vi "exec.vi"(8 "error in (no error)":errorcluster, 10 "context":refnum<class "IContextThisComponent.lvclass">, 11 "ClearError in":refnum<class "ClearError.lvclass">) -> (0 "error out":errorcluster, 2 "context 2":refnum<class "IContextThisComponent.lvclass">, 3 "ClearError out":refnum<class "ClearError.lvclass">)   [LabVIEW 2012, in "Commands.lvlib" / "ClearError.lvclass"]
uses:
  ClearError.lvclass
  IContextThisComponent/IContextThisComponent.lvclass
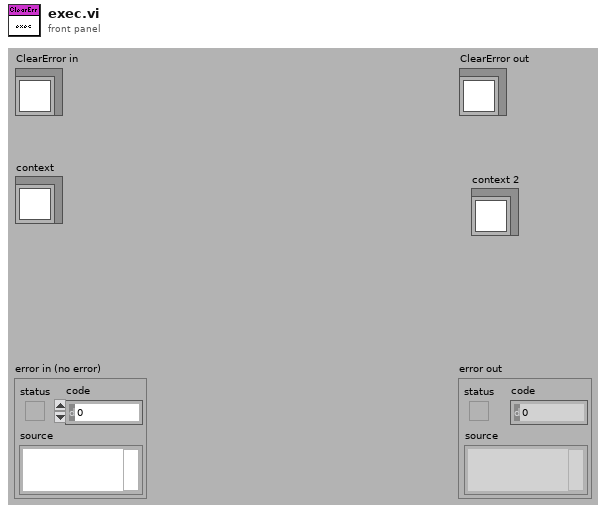
[diagram p1: front panel]
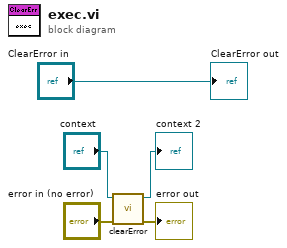
[diagram p0: block diagram]
diagram:
  n1 = call-dynamic "clearError.vi"("error in (no error)"="error in (no error)", "IContextThisComponent in"="context") -> ("error out"=→"error out":errorcluster, "IContextThisComponent out"=→"context 2":refnum<class "IContextThisComponent.lvclass">)  [unwired: 8 in]
  "ClearError out" <- "ClearError in"
